vi "脉冲测量_基于频率_单点.vi"() -> ()   [LabVIEW 2013]
uses:
  <userlib>/ArtDAQ/_SubVI/ArtDAQ_CreateCIPulseChanFreq.vi
  <userlib>/ArtDAQ/_SubVI/ArtDAQ_Read Counter Freq 1Samp.vi
panel:
  out "占空比":dbl
  out "频率":dbl
  in  "Stop":bool
  in  "计数器":string="Dev1/ctr0"
  in  "最小值":dbl=0.1 format="%0.6f"
  in  "最大值":dbl=2000000.0 format="%0.6f"
  out "错误输出":errorcluster
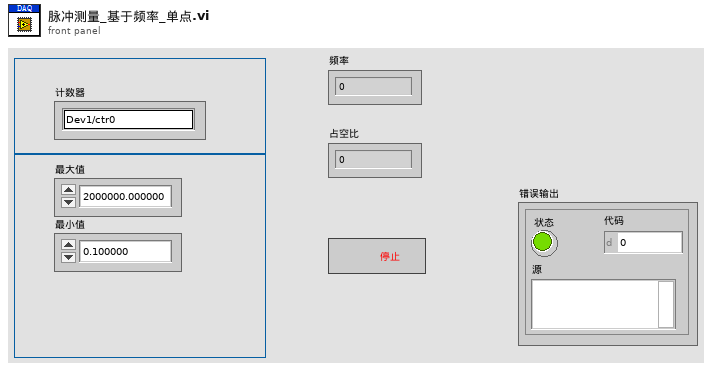
[diagram p1: front panel]
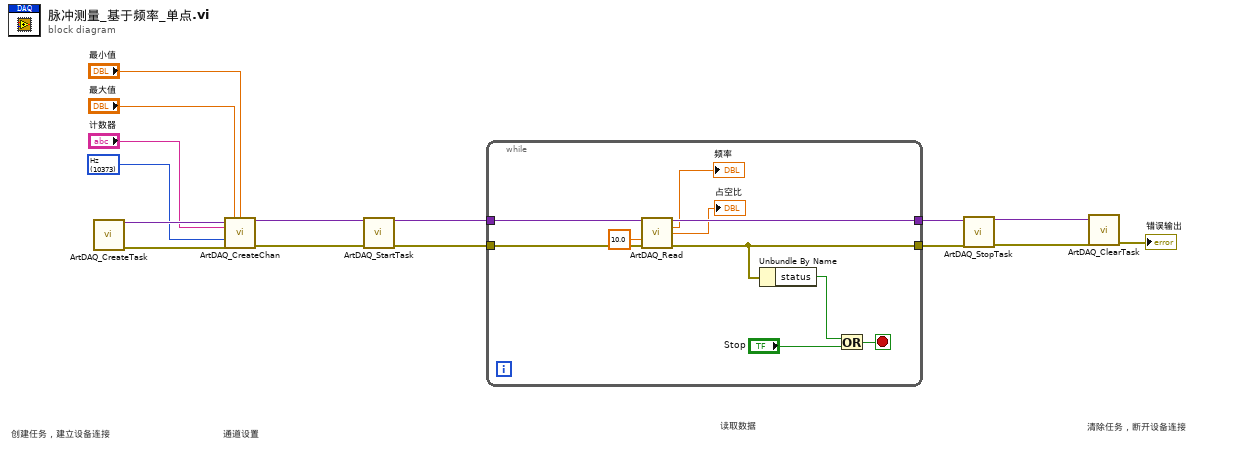
[diagram p0: block diagram]
diagram:
  w1 = 10373 items=["Hz"=10373] ("Units")
  # "清除任务，断开设备连接"
  # "读取数据"
  # "通道设置"
  # "创建任务，建立设备连接"
  n1 = call <userlib>:"ArtDAQ_CreateTask.vi"() -> ("任务句柄"=w15:variant, "错误输出"=w14:errorcluster)  [unwired: 14 in]
  n2 = call-poly <userlib>:"ArtDAQ_CreateChan.vi"("任务句柄"=w15, "最大值"="最大值", "最小值"="最小值", "计数器"="计数器", "单位"=w1, "错误输入"=w14) -> ("任务句柄"=w3:variant, "错误输出"=w2:errorcluster)  [unwired: 8 in]
  n3 = call <userlib>:"ArtDAQ_StartTask.vi"("任务句柄"=w3, "错误输入"=w2) -> ("任务句柄"=w5:variant, "错误输出"=w4:errorcluster)  [unwired: 12 in]
  n4 = while {
    tunnel: [w25] -> w7
    tunnel: [w24] -> w6
    tunnel: w5 -> [w23]
    tunnel: w4 -> [w22]
    stop <- w18 stop-if-true
    n5 = call-poly <userlib>:"ArtDAQ_Read.vi"("任务句柄"=w23, "超时s"=10.0 ("Timeout"), "错误输入"=w22) -> ("任务句柄"=w25:variant, "频率"=→"频率":dbl, "占空比"=→"占空比":dbl, "错误输出"=w24:errorcluster)  [unwired: 9 in]
    n6 = Unbundle By Name(w24) -> ("status"=w20:bool)
    n7 = Or(x=w20, y="Stop") -> (x .or. y?=w18:bool)
  }
  n8 = call <userlib>:"ArtDAQ_StopTask.vi"("任务句柄"=w7, "错误输入"=w6) -> ("任务句柄"=w12:variant, "错误输出"=w11:errorcluster)  [unwired: 12 in]
  n9 = call <userlib>:"ArtDAQ_ClearTask.vi"("任务句柄"=w12, "错误输入"=w11) -> ("错误输出"=→"错误输出":errorcluster)  [unwired: 13 in]
